vi "WPI_JoystickOpen.vi"(10 "JoystickDevice":T1) -> (3 "JoystickDevRef":T2)   [LabVIEW 2017]
doc: "Opens a reference to the joystick you specify. You must open a reference before using any other VIs on this palette. After you open a reference to the joystick, you can use the other Joystick VIs to read the button and axis values of the joystick.\n\nThis software is licensed. Open the labview\\readme\\WPI Robotics Library Open Source License.txt file for more information."
uses:
  <vilib>/Rock Robotics/WPI/Joystick/WPI_JoystickDevRef.ctl
  <vilib>/Rock Robotics/WPI/Joystick/WPI_JoystickDeviceEnum.ctl
  <vilib>/Rock Robotics/SystemInterfaces/NetworkCommunication/NetComm_UsageReport_ResourceType.ctl
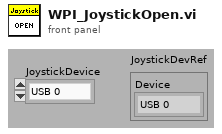
[diagram p1: front panel]
types:
  T1 = typedef "WPI_JoystickDeviceEnum.ctl" = enum16{"USB 0", "USB 1", "USB 2", "USB 3", "USB 4", "USB 5"}
  T2 = typedef "WPI_JoystickDevRef.ctl" = cluster{"Device":T1}
  T3 = typedef "NetComm_UsageReport_ResourceType.ctl" = enum8{"Controller", "Module", "Language", "CANPlugin", "Accelerometer", "ADXL345", "AnalogChannel", "AnalogTrigger", "AnalogTriggerOutput", "CANJaguar", "Compressor", "Counter", "Dashboard", "DigitalInput", "DigitalOutput", "DriverStationCIO", "DriverStationEIO", "DriverStationLCD", "Encoder", "GearTooth", "Gyro", "I2C", "Framework", "Jaguar", "Joystick", "Kinect", "KinectStick", "PIDController", "Preferences", "PWM", "Relay", "RobotDrive", "SerialPort", "Servo", "Solenoid", "SPI", "Task", "Ultrasonic", "Victor", "Button", "Command", "AxisCamera", "PCVideoServer", "SmartDashboard", "Talon", "HiTechnicColorSensor", "HiTechnicAccel", "HiTechnicCompass", "SRF08", "AnalogOutput", "Victor SP", "Talon SRX", "CAN Talon SRX", "ADXL362 Accel", "ADXRS450 Gyro", "Rev SPARK", "Mindsensors SD540", "Digital Filter", "ADIS16448", "PDP", "PCM", "PigeonIMU", "Nidec Brushless", "CTRE CANifier", "CTRE Future 0", "CTRE Future 1", "CTRE Future 2", "CTRE Future 3", "CTRE Future 4", "CTRE Future 5", "CTRE Future 6"}
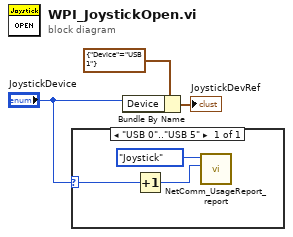
[diagram p0: block diagram]
diagram:
  n1 = case shown="\"USB 0\"..\"USB 5\"" "JoystickDevice" {
    selector: "JoystickDevice" -> [w5]
    frame "USB 0".."USB 5" {
      n2 = Increment(x=w5) -> (x+1=w4:T1)
      n3 = call <vilib>:"NetComm_UsageReport_report.vi"("Instance Number"=w4, "Resource Type"=NetComm_UsageReport_ResourceType."Joystick") -> ()  [unwired: 10 in]
    }
  }
  n4 = Bundle By Name(cluster=T2 {"Device"=enum."USB 1"} ("JoystickDevRef"), "Device"="JoystickDevice") -> (→"JoystickDevRef":T2)
